vi "OpenCVCam_TemplateMethod.vi"(8 "ErrorIn":errorcluster, 10 "CmdData":variant, 11 "OpenCVCam in":refnum<class>) -> (0 "ErrorOut":errorcluster, 2 "ReplyData":variant, 3 "OpenCVCam out":refnum<class>, 4 "Exit":bool)   [LabVIEW 2021, in "OpenCVCam.lvclass"]
uses:
  OpenCVCam.lvclass
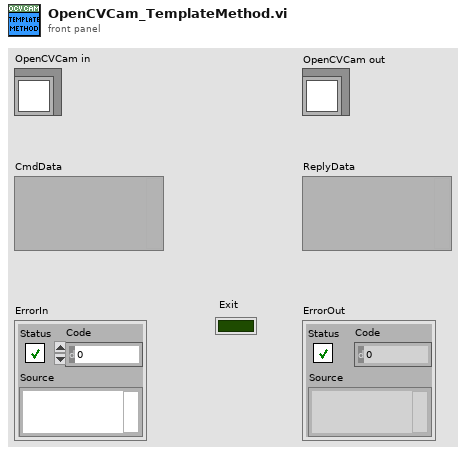
[diagram p1: front panel]
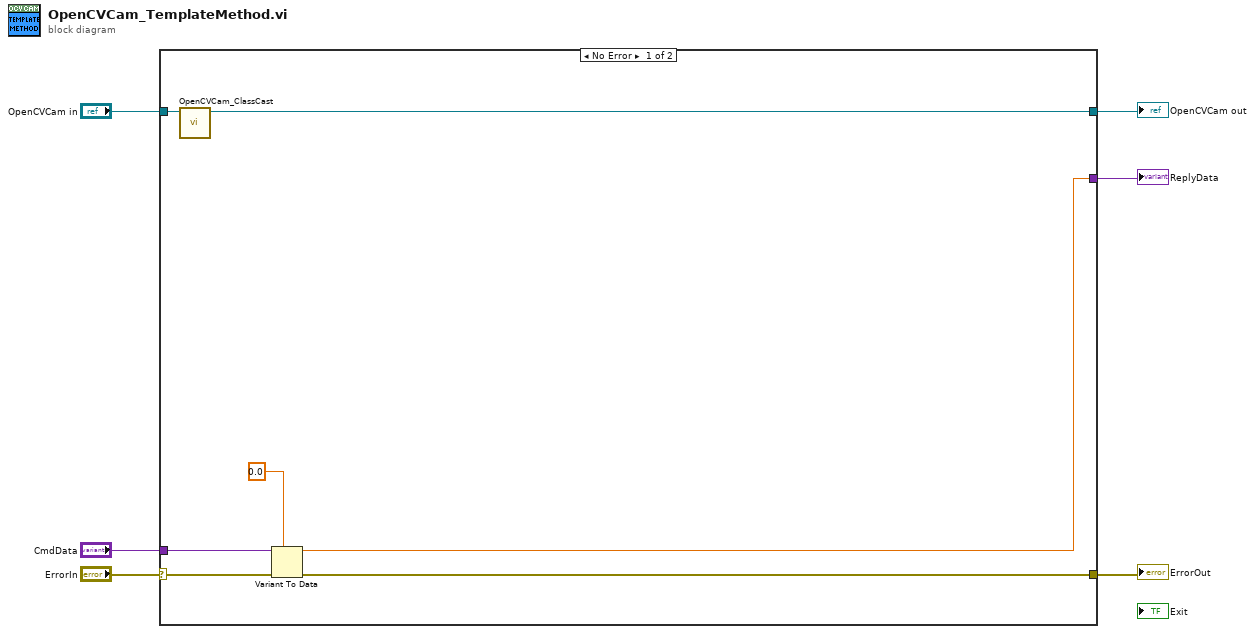
[diagram p0: block diagram]
diagram:
  n1 = case shown="No Error" "ErrorIn" {
    selector: "ErrorIn" -> [w13 w16]
    tunnel: [w9 w16] -> w5
    tunnel: [w7 w15] -> w3
    tunnel: "CmdData" -> [w11 w15]
    tunnel: "OpenCVCam in" -> [w12 w14]
    tunnel: [w10 w14] -> w1
    frame No Error {
      n2 = call "OpenCVCam_ClassCast.vi"("OpenCVCam in"=w12) -> ("OpenCVCam out"=w10:refnum<class "OpenCVCam.lvclass">)  [unwired: 10 in]
      n3 = Variant To Data(error in=w13, type=0.0 ("DummyIn"), Variant=w11) -> (data=w7:dbl, error out=w9:errorcluster)
    }
    frame Error {
    }
  }
  "ErrorOut" <- w5
  "OpenCVCam out" <- w1
  "ReplyData" <- w3
